vi "UIRef.vi"(8 "error in":errorcluster, 11 "fixed channel editor in":refnum<class "DAQmx Watchdog editor node.lvclass">) -> (0 "error out":errorcluster, 2 "VI refnum":refnum<vi>, 3 "fixed channel editor out":refnum<class "DAQmx Watchdog editor node.lvclass">)   [LabVIEW 2014, in "DAQmx Watchdog editor node.lvclass"]
uses:
  DAQmx Watchdog editor node.lvclass
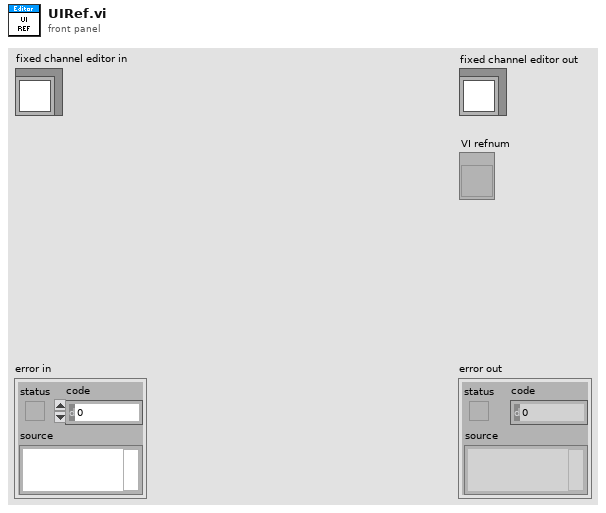
[diagram p1: front panel]
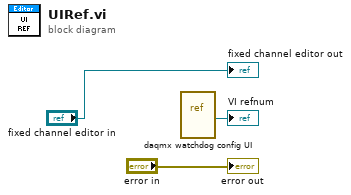
[diagram p0: block diagram]
diagram:
  n1 = vi-ref "daqmx watchdog config UI.vi"() -> (→"VI refnum":refnum<vi>)
  "error out" <- "error in"
  "fixed channel editor out" <- "fixed channel editor in"
